vi "partial.vi"(8 "input":dbl, 10 "opinon":dbl, 11 "sigmoid g(~)":dbl) -> (1 "deltaX":dbl)   [LabVIEW 2014]
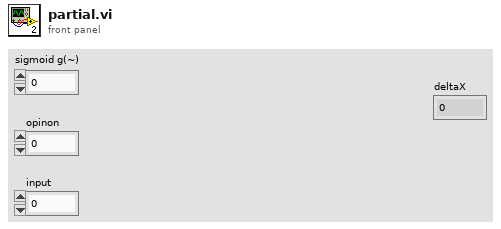
[diagram p1: front panel]
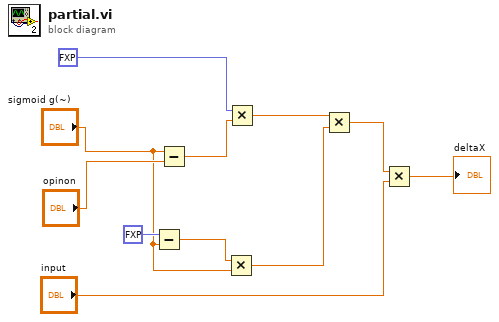
[diagram p0: block diagram]
diagram:
  n1 = Subtract(x=fxp<+/-,64,32> 1.0, y="sigmoid g(~)") -> (x-y=w7:dbl)
  n2 = Subtract(x="sigmoid g(~)", y="opinon") -> (x-y=w8:dbl)
  n3 = Multiply(x=w7, y="sigmoid g(~)") -> (x*y=w4:dbl)
  n4 = Multiply(x=fxp<+/-,64,32> 2.0, y=w8) -> (x*y=w5:dbl)
  n5 = Multiply(x=w5, y=w4) -> (x*y=w3:dbl)
  n6 = Multiply(x=w3, y="input") -> (x*y=→"deltaX":dbl)
